vi "Text Prompt.vi"(6 "Password? (F)":bool, 8 "error in (no error)":errorcluster, 9 "Default (Empty)":string, 10 "Prompt":string, 11 "CLI in":refnum<class "CLI.lvclass">) -> (0 "error out":errorcluster, 2 "Response":string, 3 "CLI out":refnum<class "CLI.lvclass">)   [LabVIEW 2020, in "neg-pkg-cli.lvlib" / "CLI.lvclass"]
uses:
  CLI.lvclass
  MGI Console/Source/Console/Console.lvclass
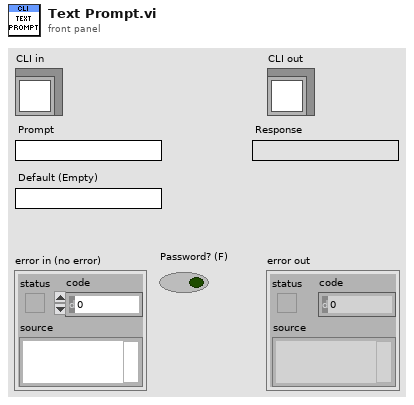
[diagram p1: front panel]
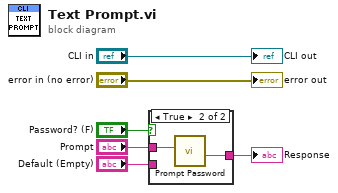
[diagram p0: block diagram]
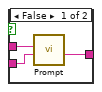
[diagram p2: hidden frame]
diagram:
  n1 = case shown="True" "Password? (F)" {
    tunnel: "Prompt" -> [w9 w11]
    tunnel: "Default (Empty)" -> [w8 _]
    tunnel: [w7 w10] -> w1
    frame False {
      n2 = call "Prompt.vi"("Default Value"=w8, "Prompt"=w9) -> ("Value"=w7:string)  [unwired: 8 in, 1 out]
    }
    frame True {
      n3 = call "Prompt Password.vi"("Prompt"=w11) -> ("Value"=w10:string)  [unwired: 9 in, 1 out]
    }
  }
  "Response" <- w1
  "error out" <- "error in (no error)"
  "CLI out" <- "CLI in"
